vi "Execute Write Read Query.vi"(0 "Driver in":refnum<class "Driver.lvclass">, 5 "Executable In":refnum<class "Executable.lvclass">, 11 "error in (no error)":errorcluster) -> (4 "Driver out":refnum<class "Driver.lvclass">, 6 "Raw Result":string, 8 "Raw Parameter Results":string[](array[string]), 10 "Executable out":refnum<class "Executable.lvclass">, 15 "error out":errorcluster)   [LabVIEW 2023, in "HAF.lvlib" / "Driver.lvclass"]
uses:
  Driver.lvclass
  Driver.lvclass/Driver.ctl
  Executable/Executable.lvclass
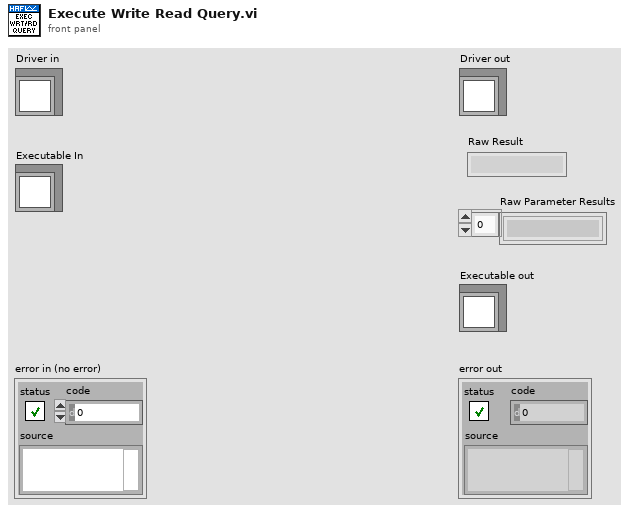
[diagram p1: front panel]
types:
  T1 = cluster{"Can Overlap":bool, "Block on Wait":bool, "Timeout":u32, "Byte Count":u32, "Parameter Count":u32}
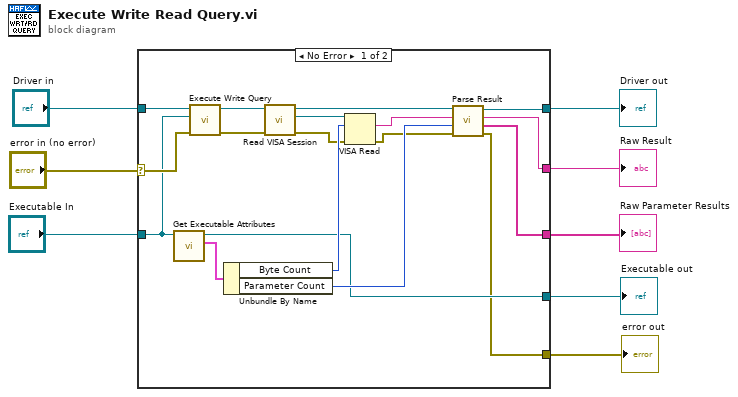
[diagram p0: block diagram]
diagram:
  n1 = case shown="No Error" "error in (no error)" {
    selector: "error in (no error)" -> [w25 w29]
    tunnel: [w9 w29] -> w7
    tunnel: [w13 w28] -> w5
    tunnel: "Driver in" -> [w26 w28]
    tunnel: "Executable In" -> [w21 w27]
    tunnel: [w12 _] -> w3
    tunnel: [w11 _] -> w2
    tunnel: [w10 w27] -> w1
    frame No Error {
      n2 = call-dynamic "Get Executable Attributes.vi"("Executable in"=w21) -> ("Executable Attributes"=w20:T1, "Executable out"=w10:refnum<class "Executable.lvclass">)  [unwired: 8 in, 1 out]
      n3 = call-dynamic "Execute Write Query.vi"("error in (no error)"=w25, "Executable In"=w21, "Driver in"=w26) -> ("error out"=w23:errorcluster, "Driver out"=w24:refnum<class "Driver.lvclass">)  [unwired: 6 in, 1 out]
      n4 = Unbundle By Name(w20) -> ("Byte Count"=w19:u32, "Parameter Count"=w15:u32)
      n5 = call-dynamic "Read VISA Session.vi"("error in (no error)"=w23, "Driver in"=w24) -> ("error out"=w18:errorcluster, "VISA Session"=w22:refnum<visa-resource-name>, "Driver out"=w17:refnum<class "Driver.lvclass">)  [unwired: 7 in]
      n6 = VISA Read(VISA resource name=w22, byte count=w19, error in (no error)=w18) -> (read buffer=w16:string, error out=w14:errorcluster)  [unwired: 2 out]
      n7 = call-dynamic "Parse Result.vi"("error in (no error)"=w14, "Number of Parameters"=w15, "Raw Result"=w16, "Driver in"=w17) -> ("error out"=w9:errorcluster, "Parameter Raw Result"=w11:string[], "Command Raw Result"=w12:string, "Driver out"=w13:refnum<class "Driver.lvclass">)  [unwired: 4 in]
    }
    frame Error {
    }
  }
  "error out" <- w7
  "Driver out" <- w5
  "Raw Result" <- w3
  "Raw Parameter Results" <- w2
  "Executable out" <- w1
